vi "Output X times.vi"(10 "?":dbl, 11 "Start":bool) -> (3 "Current #":dbl)   [LabVIEW 2012]
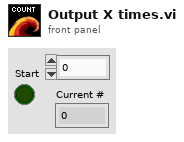
[diagram p1: front panel]
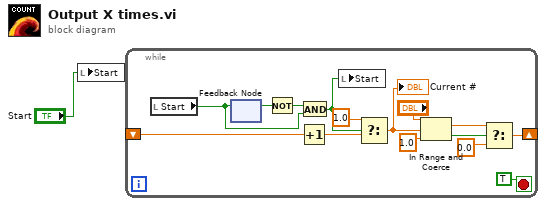
[diagram p0: block diagram]
diagram:
  n1 = local write "Start"("Start") -> ()
  n2 = while {
    shift-right: [w12] -> _
    shift-left: _ -> [w13]
    stop <- TRUE stop-if-true
    n3 = local read "Start"() -> (w5:bool)
    n4 = feedback-in #1(w5) -> ()
    n5 = feedback #1() -> (w16:bool)  [unwired: 1 in]
    n6 = Not(x=w16) -> (.not. x?=w15:bool)
    n7 = Increment(x=w13) -> (x+1=w8:dbl)
    n8 = And(x=w15, y=w5) -> (x .and. y?=w4:bool)
    n9 = local write "Start"(w4) -> ()
    n10 = Select(t=1.0, s=w4, f=w8) -> (s? t:f=w6:dbl)
    "Current #" <- w6
    n11 = In Range and Coerce(upper limit="?", x=w6, lower limit=1.0 ("upper limit")) -> (coerced(x)=w10:dbl, In Range?=w11:bool)
    n12 = Select(t=w10, s=w11, f=0.0) -> (s? t:f=w12:dbl)
  }
